vi "AppInputHdr.vi"(8 "error in (no error)":errorcluster, 11 "OutputToFileBasePlugin in":refnum<class "OutputToFileBasePlugin.lvclass">) -> (0 "error out":errorcluster, 2 "Header":string[](array[string]), 3 "OutputToFileBasePlugin out":refnum<class "OutputToFileBasePlugin.lvclass">)   [LabVIEW 2014, in "OutputToFilePlugins.lvlib" / "OutputToFileBasePlugin.lvclass"]
uses:
  OutputToFileBasePlugin.lvclass
  OutputToFileBasePlugin.lvclass/OutputToFileBasePlugin.ctl
  Accessors/Read clConfigOptions.vi
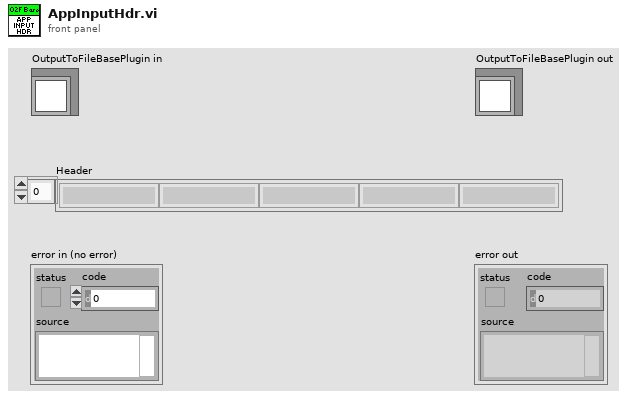
[diagram p1: front panel]
types:
  T1 = typedef "OutputToFilePlugins.lvlib/OutputToFileBasePlugin.lvclass/PmuCfgOpt.ctl" = cluster{"TIME_BASE":u64, "STN":string, "IDCODE":u16, "rdoPolRect":enum32{"Rectangular", "Polar"}, "rdoFloatInt":enum32{"Float", "Integer"}, "PHUNIT":u64, "rdoFreqDfreq":enum32{"Float", "Integer"}, "CHNAM":string[], "chkCfg2Prefix":bool}
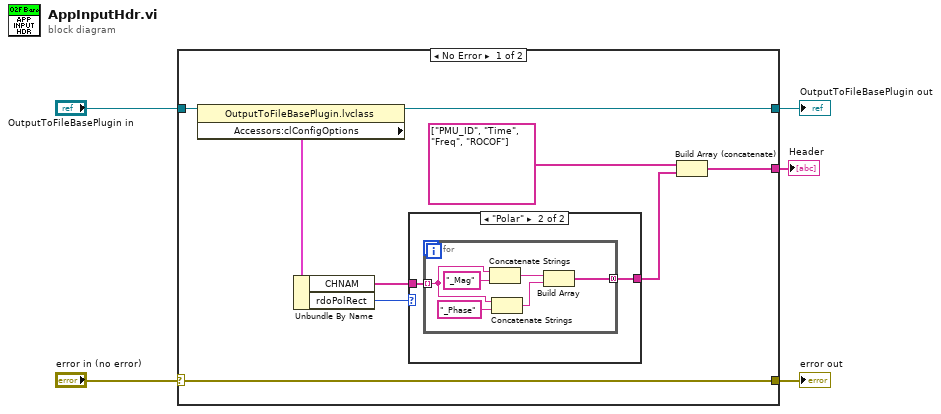
[diagram p0: block diagram]
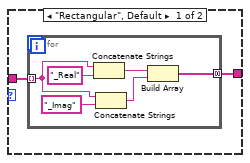
[diagram p2: hidden frame]
diagram:
  n1 = case shown="No Error" "error in (no error)" {
    selector: "error in (no error)" -> [w13 w32]
    tunnel: [w13 w32] -> w4
    tunnel: [w12 w31] -> w2
    tunnel: "OutputToFileBasePlugin in" -> [w14 w31]
    tunnel: [w7 _] -> w1
    frame No Error {
      n2 = property class="OutputToFileBasePlugin.lvclass"(reference=w14) -> (reference out=w12:refnum<class "OutputToFileBasePlugin.lvclass">, "Accessors:clConfigOptions"=w11:T1)  [unwired: 1 in, 1 out]
      n3 = Unbundle By Name(w11) -> ("CHNAM"=w10:string[], "rdoPolRect"=w8:enum32{"Rectangular", "Polar"})
      n4 = case shown="\"Polar\"" w8 {
        tunnel: w10 -> [w16 w23]
        tunnel: [w15 w24] -> w6
        frame "Rectangular", Default {
          n5 = for {
            tunnel: w16 -> [w19] mode=indexing
            tunnel: [w22] -> w15 mode=concatenating
            n6 = Concatenate Strings(w19, "_Real") -> (w17:string)
            n7 = Concatenate Strings(w19, "_Imag") -> (w18:string)
            n8 = Build Array(w17, w18) -> (w22:string[])
          }
        }
        frame "Polar" {
          n9 = for {
            tunnel: [w30] -> w24 mode=concatenating
            tunnel: w23 -> [w25] mode=indexing
            n10 = Concatenate Strings(w25, "_Mag") -> (w26:string)
            n11 = Concatenate Strings(w25, "_Phase") -> (w27:string)
            n12 = Build Array(w26, w27) -> (w30:string[])
          }
        }
      }
      n13 = Build Array (concatenate)(string[] ["PMU_ID", "Time", "Freq", "ROCOF"], w6) -> (w7:string[])
    }
    frame Error {
    }
  }
  "error out" <- w4
  "OutputToFileBasePlugin out" <- w2
  "Header" <- w1
